vi "Set Motor Power.vi"(0 "Drive Train Metrics In":T1) -> (7 "Drive Train Metrics Out":T1)   [LabVIEW 2014]
uses:
  Drive Train Metrics.ctl
  CmdFlag.ctl
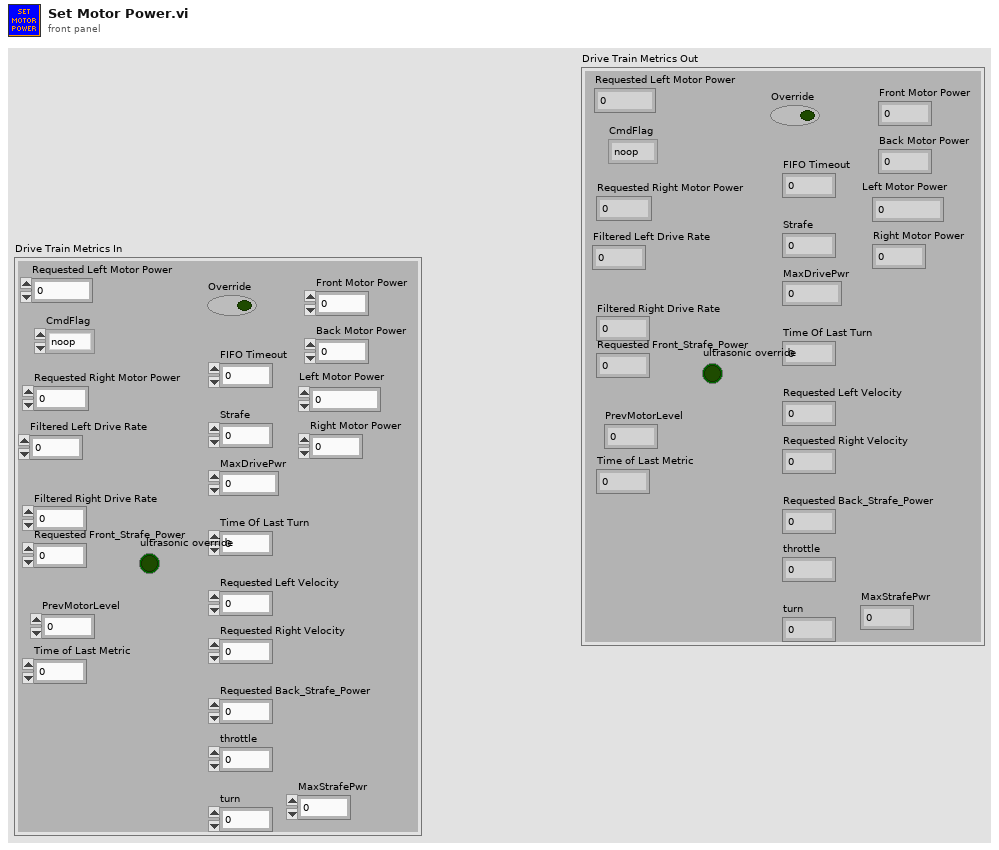
[diagram p1: front panel]
types:
  T1 = typedef "Drive Train Metrics.ctl" = cluster{"CmdFlag":T2, "Requested Right Motor Power":dbl, "Requested Left Motor Power":dbl, "Filtered Left Drive Rate":dbl, "Filtered Right Drive Rate":dbl, "Time of Last Metric":u32, "FIFO Timeout":i32, "Requested Left Velocity":dbl, "Requested Right Velocity":dbl, "throttle":dbl, "turn":dbl, "MaxDrivePwr":dbl, "Strafe":dbl, "Override":bool, "Time Of Last Turn":dbl, "Requested Front_Strafe_Power":dbl, "Requested Back_Strafe_Power":dbl, "MaxStrafePwr":dbl, "PrevMotorLevel":u8, "ultrasonic override":bool, "Left Motor Power":dbl, "Right Motor Power":dbl, "Front Motor Power":dbl, "Back Motor Power":dbl}
  T2 = typedef "CmdFlag.ctl" = enum16{"noop", "logflag", "suspend", "resume"}
  T3 = typedef "WPI_MotorControlDeviceRef.ctl" = cluster{"DeviceStatus":errorcluster, "Type":T4, "PWM":cluster{"Controller":T5, "PWM Channel":T6, "DeadBand":T7}, "CAN":cluster{"Device Number":u8, "Control Mode":T8, "Semaphore":T9, "Max Vout":dbl, "TalonSRX Control Mode":T10}, "Invert":bool, "TransformRef":T11, "InvTransformRef":T11}
  T4 = typedef "WPI_MotorControlType.ctl" = enum16{"PWM", "CAN", "CANTalonSRX"}
  T5 = typedef "FPGA_TypedefDigitalModule.ctl" = enum16{"Controller 1"}
  T6 = typedef "FPGA_DIOPWMChannel.ctl" = enum8{"PWM 0", "PWM 1", "PWM 2", "PWM 3", "PWM 4", "PWM 5", "PWM 6", "PWM 7", "PWM 8", "PWM 9", "PWM MXP 0", "PWM MXP 1", "PWM MXP 2", "PWM MXP 3", "PWM MXP 4", "PWM MXP 5", "PWM MXP 6", "PWM MXP 7", "PWM MXP 8", "PWM MXP 9", "Invalid"}
  T7 = typedef "WPI_PWMDeadband.ctl" = cluster{"Name":string, "maxPositivePwm":i32, "minPositivePwm":i32, "centerPwm":i32, "maxNegativePwm":i32, "minNegativePwm":i32, "angularRange":u16}
  T8 = typedef "WPI_CANJaguar_ControlMode.ctl" = enum8{"Percent VBus", "Current", "Speed", "Position", "Voltage"}
  T9 = typedef "Semaphore RefNum" = refnum<k1>
  T10 = typedef "WPI_CANTalonSRX_APIControlMode.ctl" = enum8{"Percent VBus", "Speed", "Position", "Slave", "Unchanged / Invalid"}
  T11 = typedef "WPI_PWMTransform_ConPane.ctl" = refnum<vi>
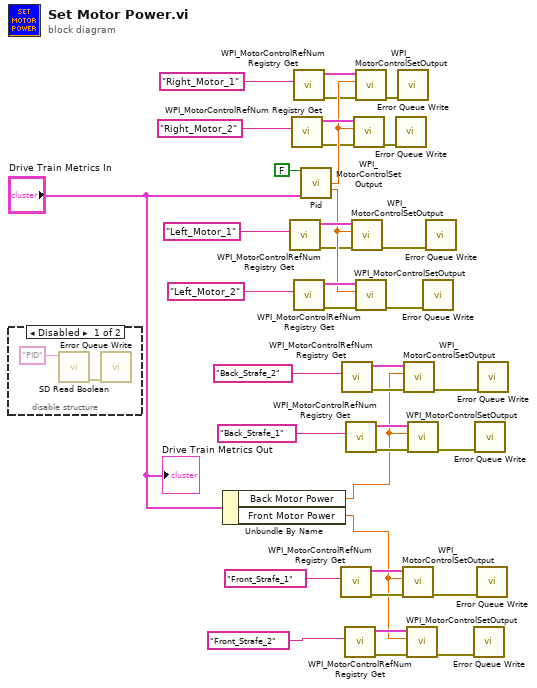
[diagram p0: block diagram]
diagram:
  n1 = disable-structure shown="Disabled" {
    frame Disabled {
      n2 = call <vilib>:"SD Read Boolean.vi"("Name"="PID") -> ("error out"=w39:errorcluster)  [unwired: 8 in, 2 out]
      n3 = call "Error Queue Write.vi"("error in (no error)"=w39) -> ()  [unwired: 11 in]
    }
    frame Enabled {
    }
  }
  n4 = Unbundle By Name("Drive Train Metrics In") -> ("Back Motor Power"=w2:dbl, "Front Motor Power"=w1:dbl)
  n5 = call <vilib>:"WPI_MotorControlRefNum Registry Get.vi"("refnum name"="Left_Motor_1") -> ("error out"=w26:errorcluster, "MotorControlDevRef"=w35:T3)  [unwired: 9 in]
  n6 = call <vilib>:"WPI_MotorControlRefNum Registry Get.vi"("refnum name"="Right_Motor_2") -> ("error out"=w22:errorcluster, "MotorControlDevRef"=w33:T3)  [unwired: 9 in]
  n7 = call <vilib>:"WPI_MotorControlRefNum Registry Get.vi"("refnum name"="Right_Motor_1") -> ("error out"=w23:errorcluster, "MotorControlDevRef"=w31:T3)  [unwired: 9 in]
  n8 = call <vilib>:"WPI_MotorControlRefNum Registry Get.vi"("refnum name"="Left_Motor_2") -> ("error out"=w27:errorcluster, "MotorControlDevRef"=w38:T3)  [unwired: 9 in]
  n9 = call "Pid.vi"("Boolean"=FALSE, "Drive Metrics"="Drive Train Metrics In") -> ("Right Motor Output"=w30:dbl, "Left Motor Output"=w29:dbl)  [unwired: 12 in]
  n10 = call <vilib>:"WPI_MotorControlRefNum Registry Get.vi"("refnum name"="Front_Strafe_1") -> ("error out"=w13:errorcluster, "MotorControlDevRef"=w15:T3)  [unwired: 9 in]
  n11 = call <vilib>:"WPI_MotorControlRefNum Registry Get.vi"("refnum name"="Back_Strafe_2") -> ("error out"=w5:errorcluster, "MotorControlDevRef"=w7:T3)  [unwired: 9 in]
  n12 = call <vilib>:"WPI_MotorControlRefNum Registry Get.vi"("refnum name"="Front_Strafe_2") -> ("error out"=w14:errorcluster, "MotorControlDevRef"=w18:T3)  [unwired: 9 in]
  n13 = call <vilib>:"WPI_MotorControlRefNum Registry Get.vi"("refnum name"="Back_Strafe_1") -> ("error out"=w6:errorcluster, "MotorControlDevRef"=w10:T3)  [unwired: 9 in]
  n14 = call <vilib>:"WPI_MotorControlSetOutput.vi"("error in (no error)"=w26, "Output"=w29, "MotorControlDevRef"=w35) -> ("error out"=w25:errorcluster)  [unwired: 6 in, 2 out]
  n15 = call <vilib>:"WPI_MotorControlSetOutput.vi"("error in (no error)"=w22, "Output"=w30, "MotorControlDevRef"=w33) -> ("error out"=w21:errorcluster)  [unwired: 6 in, 2 out]
  n16 = call <vilib>:"WPI_MotorControlSetOutput.vi"("error in (no error)"=w23, "Output"=w30, "MotorControlDevRef"=w31) -> ("error out"=w20:errorcluster)  [unwired: 6 in, 2 out]
  n17 = call <vilib>:"WPI_MotorControlSetOutput.vi"("error in (no error)"=w27, "Output"=w29, "MotorControlDevRef"=w38) -> ("error out"=w24:errorcluster)  [unwired: 6 in, 2 out]
  n18 = call "Error Queue Write.vi"("error in (no error)"=w21) -> ()  [unwired: 11 in]
  n19 = call "Error Queue Write.vi"("error in (no error)"=w20) -> ()  [unwired: 11 in]
  n20 = call <vilib>:"WPI_MotorControlSetOutput.vi"("error in (no error)"=w13, "Output"=w1, "MotorControlDevRef"=w15) -> ("error out"=w12:errorcluster)  [unwired: 6 in, 2 out]
  n21 = call <vilib>:"WPI_MotorControlSetOutput.vi"("error in (no error)"=w5, "Output"=w2, "MotorControlDevRef"=w7) -> ("error out"=w4:errorcluster)  [unwired: 6 in, 2 out]
  n22 = call <vilib>:"WPI_MotorControlSetOutput.vi"("error in (no error)"=w14, "Output"=w1, "MotorControlDevRef"=w18) -> ("error out"=w11:errorcluster)  [unwired: 6 in, 2 out]
  n23 = call <vilib>:"WPI_MotorControlSetOutput.vi"("error in (no error)"=w6, "Output"=w2, "MotorControlDevRef"=w10) -> ("error out"=w3:errorcluster)  [unwired: 6 in, 2 out]
  n24 = call "Error Queue Write.vi"("error in (no error)"=w24) -> ()  [unwired: 11 in]
  n25 = call "Error Queue Write.vi"("error in (no error)"=w25) -> ()  [unwired: 11 in]
  n26 = call "Error Queue Write.vi"("error in (no error)"=w11) -> ()  [unwired: 11 in]
  n27 = call "Error Queue Write.vi"("error in (no error)"=w3) -> ()  [unwired: 11 in]
  n28 = call "Error Queue Write.vi"("error in (no error)"=w12) -> ()  [unwired: 11 in]
  n29 = call "Error Queue Write.vi"("error in (no error)"=w4) -> ()  [unwired: 11 in]
  "Drive Train Metrics Out" <- "Drive Train Metrics In"
